vi "UHR-Fleezers Control (host) -Leonardo 04-2018 V2.vi"(0 "Tab Control":T5(tab)=enum."Trap Control (RF)") -> ()   [LabVIEW 2013] (continued)
                      n1370 = Not(x="Limits Enable") -> (.not. x?=w2097:bool)
                      n1371 = Or(x=w2098, y=w2097) -> (x .or. y?=w2099:bool)
                      n1372 = case shown="True" w2099 {
                        tunnel: w2106 -> [_ w2139]
                        tunnel: w2105 -> [_ w2130]
                        tunnel: w2095 -> [_ w2137]
                        tunnel: w2104 -> [_ w2136]
                        tunnel: w2093 -> [_ w2135]
                        tunnel: w2103 -> [_ w2134]
                        tunnel: w2088 -> [_ w2132]
                        tunnel: w2087 -> [_ w2131]
                        frame False {
                        }
                        frame True {
                          n1373 = local read "BD 1 Frequency 3 (MHz)"() -> (w2138:dbl)
                          n1374 = local read "BD 2 Frequency 3 (MHz)"() -> (w2133:dbl)
                          n1375 = local write "Trap Delta (MHz)"(w2130) -> ()
                          n1376 = property on="Initial delta (MHz)" class="DigNum (strict)"("Val(Sgnl)"=w2130) -> ()  [unwired: 2 in, 2 out]
                          n1377 = call "set RF board frequency - interlace.vi"("Board 2 Frequency Limits"=w2131, "Board 1 Frequency Limits"=w2132, "FPGA VI Reference In"=w2139, "Board 2 Frequency 3 (MHz)"=w2133, "Board 1 Frequency 3 (MHz)"=w2138, "Board 2 Frequency 2 (MHz)"=w2134, "Board 2 Frequency 1 (MHz)"=w2135, "Board 1 Frequency 2 (MHz)"=w2136, "Board 1 Frequency 1  (MHz)"=w2137) -> ()  [unwired: 1 in, 2 out]
                          n1378 = local write "BD 2 Frequency 1 (MHz)"(w2135) -> ()
                          n1379 = local write "BD 1 Frequency 1 (MHz)"(w2137) -> ()
                        }
                      }
                    }
                    frame True {
                    }
                  }
                }
                event Mouse Up {
                  n1380 = event-data() -> ("Button"=w2140:u16)  [unwired: 8 out]
                  n1381 = case shown="3" w2140 {
                    tunnel: [FALSE TRUE] -> w2141
                    frame 0, Default {
                    }
                    frame 3 {
                      n1382 = local write "Manipulating Trap"(FALSE ("Manipulating Trap")) -> ()
                    }
                  }
                }
              }
            }
          }
        }
      }
      event Mouse Move {
        n1383 = event-data() -> ()  [unwired: 6 out]
      }
    }
    n1384 = local read "Stop All"() -> (w1962:bool)
    n1385 = node-c288() -> ()  [unwired: 2 out]
  }
  n1386 = node-c288(w47) -> ()  [unwired: 1 out]
  n1387 = node-c288(w96) -> ()  [unwired: 1 out]
  n1388 = node-c288(w103) -> ()  [unwired: 1 out]
  n1389 = node-c288(i64 1 ("Period"), 1 ("Processor")) -> (w188:T25)  [unwired: 2 out]
  n1390 = timed-loop "Acquire Data" {
    tunnel: w55 -> [w2450]
    tunnel: w70 -> [w2449]
    tunnel: [w2480] -> w63
    tunnel: [w2474] -> w62
    timing: w188 -> [_]
    timing-out: [_] -> w187
    tunnel: w89 -> [w2296]
    stop <- "Stop All" stop-if-true
    (unwired) u32 0 ("Number of Elements")
    w2283 = "NI_ChannelName" ("name")
    n1391 = node-c288() -> ()  [unwired: 2 out]
    n1392 = First Call?() -> (First Call?: T/F=w2249:bool)
    n1393 = Or(x="Reset", y=w2249) -> (x .or. y?=w2250:bool)
    n1394 = local read "MCL Tracking"() -> (w2187:bool)
    n1395 = case "Reset data stream" shown="True" w2250 {
      tunnel: w2450 -> [w2600 w2608]
      tunnel: w2449 -> [w2599 w2607]
      tunnel: [w2600 w2602] -> w2185
      tunnel: [w2599 w2601] -> w2445
      frame False {
      }
      frame True {
        w2605 = TRUE ("AI to FIFO")
        n1396 = local write "Overflow (data lost)"(FALSE ("Overflow (data lost)")) -> ()
        n1397 = call "reset FPGA DMA.vi"("error in"=w2607, "FPGA VI Reference In"=w2608) -> ("error out"=w2603:errorcluster, "FPGA VI Reference Out"=w2604:T20)
        n1398 = xnode "Read/Write Control"("FPGA VI Reference In"=w2604, "error in"=w2603, "AI to FIFO"=w2605, "APD to FIFO"=w2605) -> ("FPGA VI Reference Out"=w2602:T20, "error out"=w2601:errorcluster)
      }
    }
    n1399 = Or(x="Start AOD Scan", y="Trap Raster Scan") -> (x .or. y?=w2403:bool)
    n1400 = case "Start AOM raster scan" shown="True" w2403 {
      tunnel: w2185 -> [w3341 w3352]
      tunnel: w2445 -> [w3340 w3351]
      tunnel: [w3341 w3345] -> w2184
      tunnel: [w3340 w3344] -> w2444
      frame False {
      }
      frame True {
        n1401 = case shown="True" "Restart DMA? (AOD)" {
          tunnel: [w3392 w3394] -> w3346
          tunnel: [w3391 w3393] -> w3347
          tunnel: w3352 -> [w3392 w3396]
          tunnel: w3351 -> [w3391 w3395]
          frame False {
          }
          frame True {
            n1402 = local write "Overflow (data lost)"(FALSE ("Overflow (data lost)")) -> ()
            n1403 = call "reset FPGA DMA.vi"("error in"=w3395, "FPGA VI Reference In"=w3396) -> ("error out"=w3393:errorcluster, "FPGA VI Reference Out"=w3394:T20)
          }
        }
        n1404 = local write "Trap Raster Scan"(FALSE ("Trap Raster Scan")) -> ()
        n1405 = case shown="False" "Move MCL Also?" {
          tunnel: w3347 -> [w3356 w3386]
          tunnel: w3346 -> [w3357 w3387]
          tunnel: [w3355 w3390] -> w3345
          tunnel: [w3354 w3389] -> w3344
          tunnel: "Raster to target force?" -> [w3353 w3359]
          frame False {
            w3358 = TRUE ("AI to FIFO")
            n1406 = xnode "Read/Write Control"("FPGA VI Reference In"=w3357, "error in"=w3356, "AI to FIFO"=w3358, "APD to FIFO"=w3358, "Start scan"=w3358, "Raster to target force"=w3353) -> ("FPGA VI Reference Out"=w3355:T20, "error out"=w3354:errorcluster)
          }
          frame True {
            w3383 = FALSE ("1D or 2D Scan?")
            w3388 = TRUE ("AI to FIFO")
            # "Count for MCL loop"
            # "N total cycles"
            # "N steps"
            # "V_int"
            n1407 = local read "Scan Range (nm)"() -> (w3365:dbl)
            n1408 = local read "Number of F/B Scans (AOD)"() -> (w3382:u16)
            n1409 = Sign(1:w3365) -> (0:w3364:dbl)
            n1410 = Compound Arithmetic op=MULTIPLY(w3365, "MCL Step Position Ratio", "MCL/AOM Scale Tweak") -> (w3369:dbl)
            n1411 = Negate(x=w3364) -> (-x=w3361:dbl)
            n1412 = Multiply(x=w3361, y="MCL Step Increment (V_int)") -> (x*y=w3363:dbl)
            n1413 = Divide(x=w3369, y="MCL X Cal (nm/V)") -> (x/y=w3375:dbl)
            n1414 = Multiply(x=32767.0 ("y"), y=w3375) -> (x*y=w3381:dbl)
            n1415 = local read "Total Counts (ticks)"() -> (w3366:u32)
            n1416 = local read "Cycles/step (AOD)"() -> (w3377:u64)
            n1417 = local read "Scan steps (AOD)"() -> (w3378:u64)
            n1418 = Divide(x=w3381, y=10.0) -> (x/y=w3374:dbl)
            n1419 = Divide(x=w3374, y="MCL Step Increment (V_int)") -> (x/y=w3372:dbl)
            n1420 = Absolute Value(x=w3372) -> (abs(x)=w3360:dbl)
            n1421 = Compound Arithmetic op=MULTIPLY(w3378, w3377, w3366) -> (w3373:u64)
            n1422 = local write "wait to reset values"(w3388) -> ()
            n1423 = local write "MCL Scanning"(w3388) -> ()
            n1424 = Divide(x=w3373, y=w3360) -> (x/y=w3370:dbl)
            "MCL Count" <- w3370
            n1425 = xnode "Read/Write Control"("FPGA VI Reference In"=w3387, "error in"=w3386, "Scan steps (MCL)"=w3360, "Number of scans (MCL)"=w3382, "Cycles per step (MCL)"=u64 1, "Scan freq.  increment (MCL)"=w3363, "1D or 2D Scan?"=w3383, "MCL Scan Axis"=w3383, "Cont. Scan (MCL)"=w3383, "MCL count"=w3370) -> ("FPGA VI Reference Out"=w3385:T20, "error out"=w3384:errorcluster)
            n1426 = xnode "Read/Write Control"("FPGA VI Reference In"=w3385, "error in"=w3384, "AI to FIFO"=w3388, "APD to FIFO"=w3388, "Start scan"=w3388, "Start scan (MCL)"=w3388, "Raster to target force"=w3359) -> ("FPGA VI Reference Out"=w3390:T20, "error out"=w3389:errorcluster)
          }
        }
        "Raster Scanning..." <- TRUE ("Scanning...")
      }
    }
    n1427 = And(x="Save scans", y=w2403) -> (x .and. y?=w2443:bool)
    n1428 = Compound Arithmetic op=OR("Start MCL Scan", "Confocal Image", "Confocal Linescan") -> (w2401:bool)
    n1429 = And(x="Save Data (MCL)", y=w2401) -> (x .and. y?=w2442:bool)
    n1430 = case "Start MCL raster scan" shown="True" w2401 {
      tunnel: w2184 -> [w2893 w2908]
      tunnel: w2444 -> [w2892 w2907]
      tunnel: [w2893 w2903] -> w2219
      tunnel: [w2892 w2902] -> w2218
      tunnel: [FALSE w2901] -> w2428
      tunnel: "Start MCL Scan" -> [_ w2896]
      tunnel: "Confocal Image" -> [_ w2895]
      tunnel: "Confocal Linescan" -> [_ _]
      frame False {
      }
      frame True {
        w2901 = TRUE
        n1431 = case shown="True" "Restart DMA? (MCL)" {
          tunnel: [w2953 w2955] -> w2906
          tunnel: [w2952 w2954] -> w2905
          tunnel: w2908 -> [w2953 w2958]
          tunnel: w2907 -> [w2952 w2957]
          frame False {
          }
          frame True {
            n1432 = call "reset FPGA DMA.vi"("error in"=w2957, "FPGA VI Reference In"=w2958) -> ("error out"=w2954:errorcluster, "FPGA VI Reference Out"=w2955:T20)
            n1433 = local write "Overflow (data lost)"(FALSE ("Overflow (data lost)")) -> ()
          }
        }
        n1434 = case shown="False" w2896 {
          selector: w2896 -> [_ w2912]
          tunnel: w2895 -> [w2911 _]
          tunnel: [w2911 w2912] -> w2894
          frame False {
            n1435 = property on="2D or 1D Scan" class="Bool (strict)"("Val(Sgnl)"=w2911) -> ()  [unwired: 2 in, 2 out]
            n1436 = property on="Confocal Image" class="Bool (strict)"("Value"=FALSE ("Start Confocal Map")) -> ()  [unwired: 2 in, 2 out]
          }
          frame True {
          }
        }
        n1437 = local write "MCL Scanning"(w2901) -> ()
        n1438 = local read "AO1"() -> (w2898:dbl)
        n1439 = local read "AO2"() -> (w2897:dbl)
        n1440 = case shown="True" "Center Scan" {
          tunnel: w2906 -> [w2919 w2951]
          tunnel: w2905 -> [w2918 w2950]
          tunnel: [w2917 w2949] -> w2903
          tunnel: [w2916 w2948] -> w2902
          tunnel: [w2914 w2935] -> w2900
          tunnel: [w2913 w2934] -> w2899
          tunnel: w2898 -> [w2914 w2940]
          tunnel: w2897 -> [w2913 w2943]
          tunnel: w2894 -> [_ _]
          frame False {
            w2915 = TRUE ("AI to FIFO")
            n1441 = xnode "Read/Write Control"("FPGA VI Reference In"=w2919, "error in"=w2918, "AI to FIFO"=w2915, "APD to FIFO"=w2915, "Start scan (MCL)"=w2915) -> ("FPGA VI Reference Out"=w2917:T20, "error out"=w2916:errorcluster)
          }
          frame True {
            w2947 = TRUE ("AI to FIFO")
            n1442 = local read "Scan steps (MCL)"() -> (w2926:u64)
            n1443 = local read "Scan lines (y)"() -> (w2922:u64)
            n1444 = local read "Fast Scan Dir"() -> (w2933:bool)
            n1445 = local read "Actual MCL Inc (V)"() -> (w2923:dbl)
            n1446 = Decrement(x=w2922) -> (x-1=w2921:u64)
            n1447 = Decrement(x=w2926) -> (x-1=w2925:u64)
            n1448 = Multiply(x=w2923, y=w2921) -> (x*y=w2920:dbl)
            n1449 = Divide(x=w2920, y=2.0) -> (x/y=w2930:dbl)
            n1450 = Multiply(x=w2923, y=w2925) -> (x*y=w2924:dbl)
            n1451 = Divide(x=w2924, y=2.0) -> (x/y=w2929:dbl)
            n1452 = Select(t=w2929, s=w2933, f=w2930) -> (s? t:f=w2928:dbl)
            n1453 = Select(t=w2930, s=w2933, f=w2929) -> (s? t:f=w2932:dbl)
            n1454 = Subtract(x=w2940, y=w2932) -> (x-y=w2931:dbl)
            n1455 = Subtract(x=w2943, y=w2928) -> (x-y=w2927:dbl)
            n1456 = local read "2D or 1D Scan"() -> (w2945:bool)
            n1457 = Not(x=w2933) -> (.not. x?=w2939:bool)
            n1458 = Not(x=w2945) -> (.not. x?=w2941:bool)
            n1459 = And(x=w2933, y=w2941) -> (x .and. y?=w2942:bool)
            n1460 = And(x=w2941, y=w2939) -> (x .and. y?=w2944:bool)
            n1461 = Select(t=w2943, s=w2944, f=w2927) -> (s? t:f=w2934:dbl)
            n1462 = Select(t=w2940, s=w2942, f=w2931) -> (s? t:f=w2935:dbl)
            n1463 = call "Volt to I16.vi"("Voltage In"=w2935) -> ("I16 Voltage Out"=w2938:i16)
            n1464 = call "Volt to I16.vi"("Voltage In"=w2934) -> ("I16 Voltage Out"=w2937:i16)
            n1465 = xnode "Read/Write Control"("FPGA VI Reference In"=w2951, "error in"=w2950, "AI to FIFO"=w2947, "APD to FIFO"=w2947, "Start scan (MCL)"=w2947, "AO1 (Y)"=w2938, "AO2 (X)"=w2937) -> ("FPGA VI Reference Out"=w2949:T20, "error out"=w2948:errorcluster)
          }
        }
        "Initial Y" <- w2900
        "Initial X" <- w2899
        "wait to reset values" <- w2901
      }
    }
    n1466 = local read "Trap Pos Elements/DMA read"() -> (w2292:u32)
    n1467 = local read "Trap AI Elements/DMA read"() -> (w2217:u32)
    n1468 = local read "APD Elements/DMA read"() -> (w2331:u32)
    n1469 = local read "Trap AI FIFO Depth"() -> (w2490:u32)
    n1470 = xnode "Invoke Method"("FPGA VI Reference In"=w2219, "error in"=w2218, "Number of Elements"=w2292, "Timeout (ms)"=-1) -> ("Data"=w2256:u16[], "Elements Remaining"=→"Trap Pos FIFO El Remaining":u32)  [unwired: 2 out]
    n1471 = xnode "Invoke Method"("FPGA VI Reference In"=w2219, "error in"=w2218, "Number of Elements"=w2217, "Timeout (ms)"=-1 ("Timeout")) -> ("FPGA VI Reference Out"=w2188:T20, "error out"=w2220:errorcluster, "Data"=w2216:i16[], "Elements Remaining"=w2221:u32)
    "Trap AI FIFO El. Rem." <- w2221
    n1472 = xnode "Get APD Data"("FPGA VI Reference In"=w2219, "error in"=w2218, "Number of Elements"=w2331, "Timeout (ms)"=-1) -> ("Data"=w2330:u32[], "Elements Remaining"=→"APD FIFO Elements Remaining":u32)  [unwired: 2 out]
    n1473 = Subtract(x=w2490, y=w2217) -> (x-y=w2489:u32)
    n1474 = Decimate 1D Array(w2256) -> (w2253:u16[], w2255:u16[], w2254:u16[])
    n1475 = Divide(x=w2221, y=w2489) -> (x/y=w2488:dbl)
    "Buffer Status" <- w2488
    n1476 = To Unsigned Long Integer(number=w2253) -> (unsigned 32bit integer=w2252:u32[])
    n1477 = Join Numbers(hi=w2255, lo=w2254) -> ((hi.lo)=w2251:u32[])
    n1478 = Equal?(x=w2488, y=1.0) -> (x = y?=w2486:bool)
    n1479 = Join Numbers(hi=w2252, lo=w2251) -> ((hi.lo)=w2245:u64[])
    n1480 = call "IR AOM word to freq - vec.vi"("Frequency Word In (double vec)"=w2245) -> ("Frequency Out"=w2291:dbl[])
    n1481 = case "Alert buffer overflow" shown="True" w2486 {
      frame False {
      }
      frame True {
        n1482 = call <vilib>:"Beep.vi"() -> ()  [unwired: 3 in, 9 out]
        "Overflow (data lost)" <- TRUE ("Overflow (data lost)")
      }
    }
    n1483 = Decimate 1D Array(w2291) -> (w2290:dbl[], w2289:dbl[])
    n1484 = Array Size(array=w2216) -> (size(s)=→"Waveform Chart":i32)
    n1485 = Build Array(w2290, w2289) -> (w2288:dbl[][])
    n1486 = local read "Trap Sets"() -> (w2363:u32)
    n1487 = case "Deinterlace trap data, average down PSD" shown="2" w2363 {
      tunnel: w2216 -> [w2988 w3053]
      tunnel: [w2985 w3050] -> w2356
      tunnel: [w2988 w3052] -> w2248
      tunnel: "Detector Type" -> [w2987 w3048]
      tunnel: [w2986 w3051] -> w2355
      tunnel: [w2984 w3049] -> w2461
      frame 1, Default {
        n1488 = Divide(x=w2988, y=3276.7) -> (x/y=w2989:dbl[])
        n1489 = Decimate 1D Array(w2989) -> (w2998:dbl[], w2997:dbl[], w2996:dbl[], w2995:dbl[], w2994:dbl[], w2993:dbl[], w2992:dbl[], w2991:dbl[])
        n1490 = case shown="\"IR-QPD + PSD + FB-QPD position\"" w2987 {
          tunnel: w2998 -> [w3022 w3047]
          tunnel: w2997 -> [w3021 w3046]
          tunnel: w2996 -> [w3006 w3024]
          tunnel: w2995 -> [w3007 w3034]
          tunnel: w2994 -> [w3020 w3045]
          tunnel: w2993 -> [w3019 w3044]
          tunnel: w2992 -> [w3003 w3025]
          tunnel: w2991 -> [w3002 w3023]
          tunnel: [w3001 w3031] -> w2986
          tunnel: [w3000 w3030] -> w2985
          tunnel: [w2999 w3029] -> w2984
          frame "IR-QPD + PSD + FB-QPD", Default {
            w2999 = 0  # Channel pattern
            n1491 = Divide(x=w3022, y=w3007) -> (x/y=w3009:dbl[])
            n1492 = Divide(x=w3021, y=w3007) -> (x/y=w3008:dbl[])
            n1493 = Divide(x=w3020, y=w3003) -> (x/y=w3005:dbl[])
            n1494 = Divide(x=w3019, y=w3002) -> (x/y=w3004:dbl[])
            n1495 = Build Array(w3009, w3008, w3007, w3006, w3005, w3004, w3003, w3002) -> (w3000:dbl[][])
            n1496 = Bundle("T1 Y", "T1 X", "T1 Sum", "FB Sum", "PSD Y", "PSD X", "PSD Y Sum", "PSD X Sum") -> (w3018:T42)  [unwired: 1 out]
            n1497 = Cluster To Array(cluster=w3018) -> (array=w3001:string[])
          }
          frame "IR-QPD + PSD + FB-QPD position" {
            w3029 = 3  # Channel pattern
            n1498 = Negate(x=w3025) -> (-x=w3026:dbl[])
            n1499 = Divide(x=w3047, y=w3034) -> (x/y=w3036:dbl[])
            n1500 = Divide(x=w3046, y=w3034) -> (x/y=w3035:dbl[])
            n1501 = Divide(x=w3045, y=w3025) -> (x/y=w3033:dbl[])
            n1502 = Divide(x=w3044, y=w3026) -> (x/y=w3032:dbl[])
            n1503 = Build Array(w3036, w3035, w3034, w3023, w3024, w3033, w3032, w3025) -> (w3030:dbl[][])
            n1504 = Bundle("T1 Y", "T1 X", "T1 Sum", "FB X", "FB Sum", "PSD Y", "PSD X", "PSD Y Sum") -> (w3043:T42)  [unwired: 1 out]
            n1505 = Cluster To Array(cluster=w3043) -> (array=w3031:string[])
          }
        }
      }
      frame 2 {
        n1506 = case shown="\"UCB Fleezers 052511\"" w3048 {
          tunnel: w3053 -> [w3115 w3182 w3214 w3319]
          tunnel: [w3054 w3174 w3210 w3250] -> w3052
          tunnel: [w3081 w3165 w3212 w3297] -> w3051
          tunnel: [w3080 w3129 w3201 w3264] -> w3050
          tunnel: [w3074 w3164 w3249 w3295] -> w3049
          frame "IR-QPD + PSD + FB-QPD", Default {
            w3074 = 1  # Channel pattern
            # "time average x2 the 4th signal and the 4 psd signals (detection laser)"
            # "deinterlace 3 signals from qpd"
            n1507 = Decimate 1D Array(w3115) -> (w3114:i16[], w3113:i16[], w3079:i16[], w3112:i16[], w3102:i16[], w3100:i16[], w3099:i16[], w3097:i16[])
            n1508 = call "downsample 1D array - double.vi"("Ave N"=2.0, "Array In"=w3102) -> ("Array Out"=w3101:dbl[])  [unwired: 1 out]
            n1509 = call "downsample 1D array - double.vi"("Ave N"=2.0, "Array In"=w3097) -> ("Array Out"=w3096:dbl[])  [unwired: 1 out]
            n1510 = call "downsample 1D array - double.vi"("Ave N"=2.0, "Array In"=w3099) -> ("Array Out"=w3098:dbl[])  [unwired: 1 out]
            n1511 = call "downsample 1D array - double.vi"("Ave N"=2.0, "Array In"=w3100) -> ("Array Out"=w3082:dbl[])  [unwired: 1 out]
            n1512 = Decimate 1D Array(w3114) -> (w3111:i16[], w3083:i16[])
            n1513 = Decimate 1D Array(w3113) -> (w3110:i16[], w3108:i16[])
            n1514 = Decimate 1D Array(w3112) -> (w3109:i16[], w3107:i16[])
            n1515 = Decimate 1D Array(w3079) -> (w3078:i16[], w3077:i16[])
            n1516 = Interleave 1D Arrays(w3111, w3110, w3109, w3083, w3108, w3107, w3078, w3077, w3101, w3082, w3098, w3096) -> (w3095:dbl[])
            n1517 = To Word Integer(number=w3095) -> (16bit integer=w3054:i16[])
            n1518 = Divide(x=w3095, y=3276.7) -> (x/y=w3094:dbl[])
            n1519 = Decimate 1D Array(w3094) -> (w3093:dbl[], w3092:dbl[], w3091:dbl[], w3090:dbl[], w3089:dbl[], w3088:dbl[], w3076:dbl[], w3075:dbl[], w3087:dbl[], w3086:dbl[], w3085:dbl[], w3084:dbl[])
            n1520 = Divide(x=w3093, y=w3091) -> (x/y=w3061:dbl[])
            n1521 = Divide(x=w3092, y=w3091) -> (x/y=w3060:dbl[])
            n1522 = Divide(x=w3090, y=w3088) -> (x/y=w3059:dbl[])
            n1523 = Divide(x=w3089, y=w3088) -> (x/y=w3058:dbl[])
            n1524 = Divide(x=w3087, y=w3085) -> (x/y=w3057:dbl[])
            n1525 = Divide(x=w3086, y=w3084) -> (x/y=w3056:dbl[])
            n1526 = Bundle("T1 Y", "T1 X", "T1 Sum", "T2 Y", "T2 X", "T2 Sum", "T1 FB Sum", "T2 FB Sum", "PSD Y", "PSD X", "PSD Y Sum", "PSD X Sum") -> (w3062:T43)  [unwired: 1 out]
            n1527 = Build Array(w3061, w3060, w3091, w3059, w3058, w3088, w3076, w3075, w3057, w3056, w3085, w3084) -> (w3080:dbl[][])
            n1528 = Cluster To Array(cluster=w3062) -> (array=w3081:string[])
          }
          frame "IR-QPD + PSD + FB-QPD X position" {
            w3164 = 2  # Channel pattern
            # "convert\nADC numbers\nto volts"
            # "time average x2 the 3 psd signals (detection laser)"
            # "deinterlace 3 signals from qpds"
            n1529 = Decimate 1D Array(w3182) -> (w3181:i16[], w3180:i16[], w3117:i16[], w3118:i16[], w3127:i16[], w3124:i16[], w3121:i16[], w3152:i16[])
            n1530 = Decimate 1D Array(w3181) -> (w3179:i16[], w3166:i16[])
            n1531 = call "downsample 1D array - I16.vi"("Ave N"=2.0, "Array In"=w3127) -> ("Array Out"=w3125:i16[])  [unwired: 1 in]
            n1532 = call "downsample 1D array - I16.vi"("Ave N"=2.0, "Array In"=w3124) -> ("Array Out"=w3122:i16[])  [unwired: 1 in]
            n1533 = Decimate 1D Array(w3180) -> (w3178:i16[], w3176:i16[])
            n1534 = Decimate 1D Array(w3118) -> (w3177:i16[], w3175:i16[])
            n1535 = Decimate 1D Array(w3152) -> (w3151:i16[], w3149:i16[])
            n1536 = Decimate 1D Array(w3117) -> (w3150:i16[], w3148:i16[])
            n1537 = call "downsample 1D array - I16.vi"("Ave N"=2.0, "Array In"=w3121) -> ("Array Out"=w3119:i16[])  [unwired: 1 in]
            n1538 = Interleave 1D Arrays(w3179, w3178, w3177, w3166, w3176, w3175, w3151, w3150, w3149, w3148, w3125, w3122, w3119) -> (w3174:i16[])
            n1539 = Divide(x=w3174, y=3276.7) -> (x/y=w3173:dbl[])
            n1540 = Decimate 1D Array(w3173) -> (w3172:dbl[], w3171:dbl[], w3170:dbl[], w3169:dbl[], w3168:dbl[], w3167:dbl[], w3140:dbl[], w3138:dbl[], w3137:dbl[], w3135:dbl[], w3134:dbl[], w3133:dbl[], w3130:dbl[])
            n1541 = Divide(x=w3172, y=w3170) -> (x/y=w3156:dbl[])
            n1542 = Divide(x=w3171, y=w3170) -> (x/y=w3155:dbl[])
            n1543 = Divide(x=w3169, y=w3167) -> (x/y=w3154:dbl[])
            n1544 = Divide(x=w3168, y=w3167) -> (x/y=w3153:dbl[])
            n1545 = Divide(x=w3140, y=w3138) -> (x/y=w3139:dbl[])
            n1546 = Divide(x=w3137, y=w3135) -> (x/y=w3136:dbl[])
            n1547 = Divide(x=w3134, y=w3130) -> (x/y=w3132:dbl[])
            n1548 = Negate(x=w3130) -> (-x=w3128:dbl[])
            n1549 = Divide(x=w3133, y=w3128) -> (x/y=w3131:dbl[])
            n1550 = Bundle("T1 Y", "T1 X", "T1 Sum", "T2 Y", "T2 X", "T2 Sum", "T1 FB X", "T1 FB Sum", "T2 FB X", "T2 FB Sum", "PSD Y", "PSD X", "PSD Y Sum") -> (w3157:T44)  [unwired: 1 out]
            n1551 = Build Array(w3156, w3155, w3170, w3154, w3153, w3167, w3139, w3138, w3136, w3135, w3132, w3131, w3130) -> (w3129:dbl[][])
            n1552 = Cluster To Array(cluster=w3157) -> (array=w3165:string[])
          }
          frame "UCB Fleezers 052511" {
            w3249 = 2  # Channel pattern
            n1553 = Decimate 1D Array(w3214) -> (w3247:i16[], w3246:i16[], w3195:i16[], w3213:i16[], w3187:i16[], w3209:i16[], w3208:i16[], w3192:i16[])
            n1554 = Decimate 1D Array(w3247) -> (w3245:i16[], w3232:i16[])
            n1555 = Decimate 1D Array(w3246) -> (w3244:i16[], w3243:i16[])
            n1556 = Decimate 1D Array(w3195) -> (w3189:i16[], w3188:i16[])
            n1557 = Decimate 1D Array(w3213) -> (w3194:i16[], w3193:i16[])
            n1558 = call "downsample 1D array - I16.vi"("Ave N"=2.0, "Array In"=w3187) -> ("Array Out"=w3186:i16[])  [unwired: 1 in]
            n1559 = Decimate 1D Array(w3192) -> (w3191:i16[], w3190:i16[])
            n1560 = call "downsample 1D array - I16.vi"("Ave N"=2.0, "Array In"=w3208) -> ("Array Out"=w3184:i16[])  [unwired: 1 in]
            n1561 = call "downsample 1D array - I16.vi"("Ave N"=2.0, "Array In"=w3209) -> ("Array Out"=w3185:i16[])  [unwired: 1 in]
            n1562 = Interleave 1D Arrays(w3245, w3244, w3194, w3232, w3243, w3193, w3191, w3189, w3190, w3188, w3186, w3185, w3184) -> (w3210:i16[])
            n1563 = Divide(x=w3210, y=3276.7) -> (x/y=w3239:dbl[])
            n1564 = Decimate 1D Array(w3239) -> (w3238:dbl[], w3237:dbl[], w3236:dbl[], w3235:dbl[], w3234:dbl[], w3233:dbl[], w3207:dbl[], w3205:dbl[], w3204:dbl[], w3202:dbl[], w3200:dbl[], w3197:dbl[], w3198:dbl[])
            n1565 = Divide(x=w3238, y=w3236) -> (x/y=w3219:dbl[])
            n1566 = Divide(x=w3237, y=w3236) -> (x/y=w3218:dbl[])
            n1567 = Divide(x=w3235, y=w3233) -> (x/y=w3217:dbl[])
            n1568 = Divide(x=w3234, y=w3233) -> (x/y=w3216:dbl[])
            n1569 = Divide(x=w3207, y=w3205) -> (x/y=w3206:dbl[])
            n1570 = Divide(x=w3204, y=w3202) -> (x/y=w3203:dbl[])
            n1571 = Divide(x=w3200, y=w3198) -> (x/y=w3199:dbl[])
            n1572 = Divide(x=w3197, y=w3198) -> (x/y=w3196:dbl[])
            n1573 = Build Array(w3219, w3218, w3236, w3217, w3216, w3233, w3206, w3205, w3203, w3202, w3199, w3196, w3198) -> (w3201:dbl[][])
            n1574 = Bundle("T1 Y", "T1 X", "T1 Sum", "T2 Y", "T2 X", "T2 Sum", "T1 FB X", "T2 FB Sum", "T2 FB X", "T2 FB Sum", "PSD Y", "PSD X", "PSD Sum") -> (w3220:T44)  [unwired: 1 out]
            n1575 = Cluster To Array(cluster=w3220) -> (array=w3212:string[])
          }
          frame "IR-QPD + PSD + FB-QPD XY positions" {
            w3295 = 4  # Channel pattern
            # "time average x2 the 3 psd signals (detection laser)"
            # "deinterlace 3 signals from qpds"
            n1576 = Decimate 1D Array(w3319) -> (w3318:i16[], w3317:i16[], w3296:i16[], w3316:i16[], w3262:i16[], w3308:i16[], w3307:i16[], w3284:i16[])
            n1577 = Decimate 1D Array "QPD Y"(w3318) -> (w3315:i16[], w3298:i16[])
            n1578 = call "downsample 1D array - double.vi"("Ave N"=2.0, "Array In"=w3308) -> ("Array Out"=w3283:dbl[])  [unwired: 1 out]
            n1579 = call "downsample 1D array - double.vi"("Ave N"=2.0, "Array In"=w3307) -> ("Array Out"=w3282:dbl[])  [unwired: 1 out]
            n1580 = Decimate 1D Array "Feedback Sum"(w3296) -> (w3280:i16[], w3278:i16[])
            n1581 = Decimate 1D Array "Feedback Y"(w3262) -> (w3261:i16[], w3260:i16[])
            n1582 = Decimate 1D Array "Feedback X"(w3284) -> (w3281:i16[], w3279:i16[])
            n1583 = Decimate 1D Array "QPD Sum"(w3316) -> (w3313:i16[], w3311:i16[])
            n1584 = Decimate 1D Array "QPD X"(w3317) -> (w3314:i16[], w3312:i16[])
            n1585 = Interleave 1D Arrays(w3315, w3314, w3313, w3298, w3312, w3311, w3261, w3281, w3280, w3260, w3279, w3278, w3283, w3282) -> (w3306:dbl[])
            n1586 = To Word Integer(number=w3306) -> (16bit integer=w3250:i16[])
            n1587 = Divide(x=w3306, y=3276.7) -> (x/y=w3305:dbl[])
            n1588 = Decimate 1D Array(w3305) -> (w3304:dbl[], w3303:dbl[], w3302:dbl[], w3301:dbl[], w3300:dbl[], w3299:dbl[], w3257:dbl[], w3271:dbl[], w3255:dbl[], w3256:dbl[], w3269:dbl[], w3253:dbl[], w3267:dbl[], w3265:dbl[])
            n1589 = Divide(x=w3304, y=w3302) -> (x/y=w3288:dbl[])
            n1590 = Divide(x=w3303, y=w3302) -> (x/y=w3287:dbl[])
            n1591 = Divide(x=w3301, y=w3299) -> (x/y=w3286:dbl[])
            n1592 = Divide(x=w3300, y=w3299) -> (x/y=w3285:dbl[])
            n1593 = Divide(x=w3257, y=w3255) -> (x/y=w3254:dbl[])
            n1594 = Divide(x=w3271, y=w3255) -> (x/y=w3270:dbl[])
            n1595 = Divide(x=w3256, y=w3253) -> (x/y=w3252:dbl[])
            n1596 = Divide(x=w3269, y=w3253) -> (x/y=w3268:dbl[])
            n1597 = Negate(x=w3265) -> (-x=w3263:dbl[])
            n1598 = Divide(x=w3267, y=w3263) -> (x/y=w3266:dbl[])
            n1599 = Bundle("T1 Y", "T1 X", "T1 Sum", "T2 Y", "T2 X", "T2 Sum", "T1 FB Y", "T1 FB X", "T1 FB Sum", "T2 FB Y", "T2 FB X", "T2 FB Sum", "PSD X", "PSD Y Sum") -> (w3251:T45)  [unwired: 1 out]
            n1600 = Build Array(w3288, w3287, w3302, w3286, w3285, w3299, w3254, w3270, w3255, w3252, w3268, w3253, w3266, w3265) -> (w3264:dbl[][])
            n1601 = Cluster To Array(cluster=w3251) -> (array=w3297:string[])
          }
        }
      }
    }
    "AI labels" <- w2355
    n1602 = xnode "Read/Write Control"("FPGA VI Reference In"=w2188) -> ("FPGA VI Reference Out"=w2181:T20, "BD1 Frequency Out 1"=w2202:u64)  [unwired: 1 in, 1 out]
    n1603 = local read "BD 1 Frequency 2 (MHz)"() -> (w2193:dbl)
    n1604 = To Double Precision Float(number=w2202) -> (double precision float=w2199:dbl)
    n1605 = Multiply(x=49125000.0, y=6.0) -> (x*y=w2198:dbl)
    n1606 = Multiply(x=w2199, y=w2198) -> (x*y=w2196:dbl)
    n1607 = Scale By Power Of 2(n=-48, x=w2196) -> (x*2^n=w2195:dbl)
    n1608 = local read "Dynamic Force FB"() -> (w2192:bool)
    n1609 = local read "Trap Pos. FB ON"() -> (w2191:bool)
    n1610 = Divide(x=w2195, y=1000000.0) -> (x/y=w2186:dbl)
    n1611 = case shown="True" w2187 {
      tunnel: w2186 -> [_ w2577]
      tunnel: w2184 -> [_ w2564]
      frame False {
      }
      frame True {
        n1612 = local read "AOM X Cal (nm/MHz)"() -> (w2574:dbl)
        n1613 = local read "Zero T1 position"() -> (w2576:dbl)
        n1614 = Subtract(x=w2577, y=w2576) -> (x-y=w2575:dbl)
        n1615 = Multiply(x=w2575, y=w2574) -> (x*y=w2573:dbl)
        n1616 = local read "MCL X Cal (nm/V)"() -> (w2570:dbl)
        n1617 = Multiply(x=w2573, y="Tracking factor") -> (x*y=w2571:dbl)
        n1618 = local read "Zero MCL x position"() -> (w2569:dbl)
        n1619 = Divide(x=w2571, y=w2570) -> (x/y=w2568:dbl)
        n1620 = Add(x=w2569, y=w2568) -> (x+y=w2561:dbl)
        "Current MCL (V)" <- w2561
        n1621 = Multiply(x=w2561, y=32767.0) -> (x*y=w2565:dbl)
        n1622 = Divide(x=w2565, y=10.0) -> (x/y=w2562:dbl)
        n1623 = To Word Integer(number=w2562) -> (16bit integer=w2563:i16)
        n1624 = xnode "Read/Write Control"("FPGA VI Reference In"=w2564, "AO2 (X)"=w2563) -> ()  [unwired: 1 in, 2 out]
      }
    }
    n1625 = Subtract(x=w2193, y=w2186) -> (x-y=w2182:dbl)
    "Current deltaFreq" <- w2182
    n1626 = Compound Arithmetic op=AND(w2192, w2191, "Real time offset \ncorrection for setpoint") -> (w2189:bool)
    n1627 = case shown="True" w2189 {
      tunnel: w2182 -> [_ w2580]
      tunnel: w2181 -> [_ w2579]
      frame False {
      }
      frame True {
        n1628 = local read "T1 kappa_x (pN/nm)"() -> (w2588:dbl)
        n1629 = local read "T1 alpha_x (nm/V)"() -> (w2589:dbl)
        n1630 = local read "Negate offset difference"() -> (w2590:bool)
        n1631 = local read "Offset file step size"() -> (w2598:dbl)
        n1632 = Multiply(x="Target Force (pN)", y=2.0) -> (x*y=w2586:dbl)
        n1633 = local read "Setpoint offset\nCorrection values"() -> (w2595:dbl[])
        n1634 = Divide(x=w2580, y=w2598) -> (x/y=w2597:dbl)
        n1635 = Select(t=-1, s=w2590, f=1) -> (s? t:f=w2591:i32)
        n1636 = To Long Integer(number=w2597) -> (32bit integer=w2596:i32)
        n1637 = Multiply(x=w2589, y=w2588) -> (x*y=w2585:dbl)
        n1638 = Divide(x=w2586, y=w2585) -> (x/y=w2584:dbl)
        n1639 = Index Array(array=w2595, index=w2596) -> (element=w2594:dbl)
        n1640 = Multiply(x=w2591, y=w2594) -> (x*y=w2583:dbl)
        n1641 = Add(x=w2584, y=w2583) -> (x+y=w2582:dbl)
        n1642 = To Fixed-Point(number=w2582) -> (fixed-point=w2578:fxp<+/-,16,1>)  [unwired: 1 in]
        "Actual setpoint" <- w2578
        n1643 = xnode "Read/Write Control"("FPGA VI Reference In"=w2579, "Trap Pos. FB SP"=w2578) -> ()  [unwired: 1 in, 2 out]
      }
    }
    n1644 = case shown="True" "Take full offset\n data for display" {
      tunnel: [w2547 w2553] -> w2380
      tunnel: [w2546 w2552] -> w2378
      tunnel: w2182 -> [_ w2559]
      frame False {
        n1645 = Divide(x="T2 offset_x (mV)", y=1000.0) -> (x/y=w2546:dbl)
        n1646 = Divide(x="T1 offset_x (mV)", y=1000.0) -> (x/y=w2547:dbl)
      }
      frame True {
        n1647 = local read "Offset Values"() -> (w2560:T14)
        n1648 = local read "Offset file step size"() -> (w2558:dbl)
        n1649 = Unbundle By Name(w2560) -> ("Trap 1X offset"=w2555:dbl[], "Trap 2X offset"=w2554:dbl[])
        n1650 = Divide(x=w2559, y=w2558) -> (x/y=w2557:dbl)
        n1651 = To Long Integer(number=w2557) -> (32bit integer=w2556:i32)
        n1652 = Index Array(array=w2555, index=w2556) -> (element=w2553:dbl)
        n1653 = Index Array(array=w2554, index=w2556) -> (element=w2552:dbl)
      }
    }
    n1654 = Decimate 1D Array(w2330) -> (w2353:u32[], w2298:u32[])
    n1655 = local read "DMA Update Period (s)"() -> (w2364:dbl)
    n1656 = local read "BD 1 Frequency 2 (MHz)"() -> (w2240:dbl)
    n1657 = local read "BD 1 Frequency 1 (MHz)"() -> (w2241:dbl)
    n1658 = Build Array(w2353, w2298) -> (w2425:u32[][])
    n1659 = local read "Data Period (s)"() -> (w2343:dbl)
    n1660 = Decimate 1D Array(w2248) -> (w2271:i16[], w2270:i16[], w2268:i16[], w2267:i16[])  [unwired: 9 out]
    n1661 = To Double Precision Float(number=w2425) -> (double precision float=w2426:dbl[][])
    n1662 = local read "APD Integration Time (s)"() -> (w2311:dbl)
    n1663 = Divide(x=w2271, y=w2270) -> (x/y=w2272:dbl[])
    n1664 = Divide(x=w2268, y=w2267) -> (x/y=w2269:dbl[])
    n1665 = feedback #1(0.0) -> (w2285:dbl)
    n1666 = Add(x=w2364, y=w2285) -> (x+y=w2463:dbl)
    n1667 = feedback-in #1(w2463) -> ()
    n1668 = local read "AOM X Cal (nm/MHz)"() -> (w2238:dbl)
    n1669 = To Time Stamp(1:w2285) -> (0:w2284:timestamp)
    n1670 = Split 1D Array(array=w2272, index="N El. to Ave.") -> (second subarray=w2275:dbl[])  [unwired: 1 out]
    n1671 = Split 1D Array(array=w2269, index="N El. to Ave.") -> (second subarray=w2274:dbl[])  [unwired: 1 out]
    n1672 = local read "Trap X AI1 (DMA)"() -> (w2273:T13)
    n1673 = Multiply(x=w2343, y="Trap Disp. Downsample") -> (x*y=w2286:dbl)
    "Display Period (s)" <- w2286
    n1674 = Bundle("BD 1 Frequency 1 (MHz)"=w2241, "BD 1 Frequency 2 (MHz)"=w2240) -> (w2242:T46)  [unwired: 1 out]
    n1675 = for "Trap AI" {
      tunnel: [w2983] -> w2457 mode=indexing
      tunnel: w2284 -> [w2973]
      tunnel: "Trap Disp. Downsample" -> [w2981]
      tunnel: w2356 -> [w2979] mode=indexing
      tunnel: w2343 -> [w2978]
      tunnel: w2355 -> [w2977] mode=indexing
      tunnel: w2283 -> [w2976]
      tunnel: [w2975] -> w2322 mode=indexing
      tunnel: w2286 -> [w2974]
      n1676 = Bundle By Name("Y"=w2979, "dt"=w2978) -> (w2980:waveform(dbl))  [unwired: 1 out]
      n1677 = Set Waveform Attribute(5:w2977, 6:w2976, 7:w2980) -> (3:w2975:waveform(dbl))  [unwired: 1 in, 2 out]
      n1678 = call "downsample 1D array - double.vi"("Ave N"=w2981, "Array In"=w2979) -> ("Array Out"=w2982:dbl[])  [unwired: 1 out]
      n1679 = Bundle By Name(cluster=w2975, "t0"=w2973, "Y"=w2982, "dt"=w2974) -> (w2983:waveform(dbl))
    }
    n1680 = call-poly <vilib>:"Mean.vi"("X"=w2274) -> ("mean"=w2262:dbl)  [unwired: 1 out]
    n1681 = call-poly <vilib>:"Mean.vi"("X"=w2275) -> ("mean"=w2263:dbl)  [unwired: 1 out]
    n1682 = Cluster To Array(cluster=w2242) -> (array=w2239:dbl[])
    n1683 = Reciprocal(x=w2286) -> (1/x=→"Trap Disp. Freq. (Hz)":dbl)
    n1684 = local read "Data points/scans (MCL)"() -> (w2437:dbl)
    n1685 = To Fixed-Point(number=w2262) -> (fixed-point=w2260:fxp<+/-,16,1>)  [unwired: 1 in]
    n1686 = To Fixed-Point(number=w2263) -> (fixed-point=w2261:fxp<+/-,16,1>)  [unwired: 1 in]
    n1687 = Bundle("Trap 1 Pos.", "Trap 2 Pos.") -> (w2282:cluster{string, string})  [unwired: 1 out]
    n1688 = Bundle By Name(cluster=w2273, "Set 1"=w2261, "Set 2"=w2260) -> (→"Trap X AI1 (DMA)":T13)
    n1689 = Cluster To Array(cluster=w2282) -> (array=w2279:string[])
    n1690 = for "Trap Position" {
      tunnel: w2288 -> [w2621] mode=indexing
      tunnel: "Trap Disp. Downsample" -> [w2620]
      tunnel: w2286 -> [w2618]
      tunnel: w2284 -> [w2617]
      tunnel: w2283 -> [w2615]
      tunnel: w2279 -> [w2614] mode=indexing
      tunnel: [w2613] -> w2237 mode=indexing
      tunnel: w2239 -> [w2611] mode=indexing
      tunnel: w2238 -> [w2609]
      n1691 = call "downsample 1D array - double.vi"("Ave N"=w2620, "Array In"=w2621) -> ("Array Out"=w2619:dbl[])  [unwired: 1 out]
      n1692 = Subtract(x=w2619, y=w2611) -> (x-y=w2612:dbl[])
      n1693 = Multiply(x=w2609, y=w2612) -> (x*y=w2610:dbl[])
      n1694 = Bundle By Name("Y"=w2610, "dt"=w2618, "t0"=w2617) -> (w2616:waveform(dbl))  [unwired: 1 out]
      n1695 = Set Waveform Attribute(5:w2614, 6:w2615, 7:w2616) -> (3:w2613:waveform(dbl))  [unwired: 1 in, 2 out]
    }
    "Trap Positions" <- w2237
    n1696 = Bundle("APD 1", "APD 2") -> (w2456:cluster{string, string})  [unwired: 1 out]
    n1697 = Cluster To Array(cluster=w2456) -> (array=w2453:string[])
    n1698 = for "APD" {
      tunnel: w2426 -> [w2962] mode=indexing
      tunnel: w2311 -> [w2970]
      tunnel: [w2966] -> w2318 mode=indexing
      tunnel: "APD Disp. Scale" -> [w2967]
      tunnel: w2283 -> [w2965]
      tunnel: w2453 -> [w2964] mode=indexing
      tunnel: "APD Disp. Downsample" -> [w2960]
      tunnel: [w2963] -> w2452
      tunnel: w2284 -> [w2959]
      n1699 = call "integrate 1D array interval - double.vi"("Ave N"=w2960, "Array In"=w2962) -> ("Array Out"=w2961:dbl[])  [unwired: 1 out]
      n1700 = Multiply(x=w2970, y=w2960) -> (x*y=w2963:dbl)
      n1701 = Divide(x=w2961, y=w2967) -> (x/y=w2968:dbl[])
      n1702 = Bundle By Name("t0"=w2959, "Y"=w2968, "dt"=w2963) -> (w2969:waveform(dbl))  [unwired: 1 out]
      n1703 = Set Waveform Attribute(5:w2964, 6:w2965, 7:w2969) -> (3:w2966:waveform(dbl))  [unwired: 1 in, 2 out]
    }
    "APD Display Period (s)" <- w2452
    n1704 = Reciprocal(x=w2452) -> (1/x=→"APD Display Freq. (Hz)":dbl)
    n1705 = local read "Display Period (s)"() -> (w2342:dbl)
    n1706 = Increment(x=w2437) -> (x+1=w2438:dbl)
    n1707 = Index Array(array=w2237, index=0) -> (element=w2235:waveform(dbl))
    n1708 = To Double Precision Float(number=w2353) -> (double precision float=w2352:dbl[])
    n1709 = feedback #2(w2438) -> (w2441:dbl)
    n1710 = Select(t=0, s=w2428, f=w2441) -> (s? t:f=w2434:dbl)
    n1711 = Array Size(array=w2352) -> (size(s)=w2440:i32)
    n1712 = Add(x=w2440, y=w2434) -> (x+y=w2435:dbl)
    n1713 = Unbundle By Name(w2235) -> ("Y"=w2233:dbl[])
    n1714 = feedback #3(w2353) -> (w2424:u32[])
    n1715 = Build Array (concatenate)(w2424, w2353) -> (w2421:u32[])
    n1716 = feedback #4(w2298) -> (w2317:u32[])
    n1717 = Divide(x="Bead Sep. Int. Time (s)", y=w2342) -> (x/y=w2231:dbl)
    n1718 = Build Array (concatenate)(w2317, w2298) -> (w2316:u32[])
    n1719 = Greater?(x=w2435, y=w2437) -> (0:w2436:bool)
    n1720 = feedback #5(w2233) -> (w2234:dbl[])
    n1721 = Build Array (concatenate)(w2233, w2234) -> (w2232:dbl[])
    n1722 = Select(t=w2434, s=w2436, f=w2435) -> (s? t:f=w2433:dbl)
    n1723 = feedback-in #2(w2433) -> ()
    n1724 = Array Size(array=w2421) -> (size(s)=w2418:i32)
    n1725 = Array Size(array=w2353) -> (size(s)=w2420:i32)
    n1726 = local read "MCL Scanning"() -> (w2431:bool)
    n1727 = local read "APD Integration Time (s)"() -> (w2325:dbl)
    n1728 = Build Array (concatenate)(w2318, w2457) -> (w2320:waveform(dbl)[])
    "All Signals" <- w2320
    n1729 = Split 1D Array(array=w2232, index=w2231) -> (first subarray=w2225:dbl[])  [unwired: 1 out]
    n1730 = feedback-in #5(w2225) -> ()
    n1731 = Multiply(x=w2420, y="APD Ave N") -> (x*y=w2419:dbl)
    n1732 = Greater?(x=w2418, y=w2419) -> (0:w2422:bool)
    n1733 = Not(x=w2436) -> (.not. x?=w2430:bool)
    n1734 = To Double Precision Float(number=w2298) -> (double precision float=w2297:dbl[])
    n1735 = call-poly <vilib>:"Mean.vi"("X"=w2225) -> ("mean"=w2224:dbl)  [unwired: 1 out]
    "Mean T1 Position (nm)" <- w2224
    n1736 = Subtract(x=w2225, y=w2224) -> (x-y=w2230:dbl[])
    n1737 = Square(x=w2230) -> (x^2=w2229:dbl[])
    n1738 = And(x=w2430, y=w2431) -> (x .and. y?=w2432:bool)
    n1739 = call-poly <vilib>:"Mean.vi"("X"=w2229) -> ("mean"=w2228:dbl)  [unwired: 1 out]
    n1740 = case shown="True" w2422 {
      tunnel: w2421 -> [w2743 w2750]
      tunnel: [w2743 w2748] -> w2369
      tunnel: w2419 -> [_ w2745]
      tunnel: w2418 -> [_ w2749]
      tunnel: w2316 -> [w2742 w2747]
      tunnel: [w2742 w2744] -> w2313
      frame False {
      }
      frame True {
        n1741 = Subtract(x=w2749, y=w2745) -> (x-y=w2746:dbl)
        n1742 = Array Subset(array=w2750, index=w2746, length=w2745) -> (w2748:u32[])
        n1743 = Array Subset(array=w2747, index=w2746, length=w2745) -> (w2744:u32[])
      }
    }
    n1744 = feedback-in #3(w2369) -> ()
    n1745 = feedback-in #4(w2313) -> ()
    n1746 = Or(x=w2432, y=w2428) -> (x .or. y?=w2429:bool)
    n1747 = Square Root(x=w2228) -> (sqrt(x)=w2227:dbl)
    n1748 = Equal?(x="Tab Control 6", y=T36."High Res Display") -> (x = y?=w2359:bool)
    n1749 = Multiply(x="APD Disp. Scale", y=w2318) -> (x*y=w2327:waveform(dbl)[])
    n1750 = Multiply(x="APD Disp. Downsample", y=w2325) -> (x*y=w2323:dbl)
    n1751 = Multiply(x=10.0, y=w2227) -> (x*y=→"Trap 1 Position RMS (A)":dbl)
    n1752 = Divide(x=w2327, y=w2323) -> (x/y=w2295:waveform(dbl)[])
    n1753 = Index Array(array=w2295, index=0) -> (element=w2305:waveform(dbl))
    n1754 = case "For computing FFTs for display" shown="True" "Compute FFT" {
      tunnel: w2322 -> [_ w3425]
      frame False {
      }
      frame True {
        n1755 = Build Array("FFT 1 Choice 1", "FFT 1 Choice 2", "FFT 2 Choice 1", "FFT 2 Choice 2") -> (w3418:u16[])
        n1756 = Array Size(array=w3425) -> (size(s)=w3424:i32)
        n1757 = feedback-in #6(w3418) -> ()
        n1758 = feedback #6(u16[] [100, 100, 100, 100]) -> (w3419:u16[])
        n1759 = feedback-in #7("# Spectra to Ave.") -> ()
        n1760 = feedback #7("# Spectra to Ave.") -> (w3416:dbl)
        n1761 = Not Equal?(x="# Spectra to Ave.", y=w3416) -> (x != y?=w3415:bool)
        n1762 = Not Equal?(x=w3418, y=w3419) -> (x != y?=w3417:bool)
        n1763 = feedback #8(1.0) -> (w3402:dbl)
        n1764 = Compound Arithmetic op=OR("Reset FFT", w3417, w3415) -> (w3400:bool)
        n1765 = Select(t=1.0, s=w3400, f=w3402) -> (s? t:f=w3404:dbl)
        n1766 = Greater?(x=w3404, y="# Spectra to Ave.") -> (0:w3423:bool)
        n1767 = Increment(x=w3404) -> (x+1=w3403:dbl)
        n1768 = feedback-in #8(w3403) -> ()
        n1769 = local read "DMA Update Period (s)"() -> (w3398:dbl)
        n1770 = Multiply(x="# Spectra to Ave.", y=w3398) -> (x*y=→"Ave. Time (s)":dbl)
        n1771 = Build Array(cluster{"f0":dbl, "df":dbl, "magnitude":dbl[]} {"f0"=0.0, "df"=0.0, "magnitude"=[]} ("PSD")) -> (w3407:cluster{"f0":dbl, "df":dbl, "magnitude":dbl[]}[])
        n1772 = Build Array(w3407, w3407, w3407, w3407) -> (w3409:T47)
        n1773 = feedback #9(w3409) -> (w3414:T47)
        n1774 = for {
          N: 4 -> [_]
          tunnel: w3418 -> [w3447] mode=indexing
          tunnel: w3425 -> [w3448]
          tunnel: w3424 -> [w3450]
          tunnel: w3400 -> [w3443]
          tunnel: w3423 -> [w3442]
          tunnel: "# Spectra to Ave." -> [w3441]
          tunnel: [w3440] -> w3413 mode=indexing
          tunnel: w3414 -> [w3445] mode=indexing
          tunnel: [w3444] -> w3401 mode=indexing
          tunnel: w3404 -> [w3439]
          n1775 = Less?(x=w3447, y=w3450) -> (x < y?=w3449:bool)
          n1776 = Index Array(array=w3448, index=w3447) -> (element=w3446:waveform(dbl))
          n1777 = case shown="True" w3449 {
            tunnel: w3446 -> [_ w3467]
            tunnel: w3445 -> [w3452 w3465]
            tunnel: [w3452 w3453] -> w3444
            tunnel: w3443 -> [_ w3464]
            tunnel: w3442 -> [_ w3457]
            tunnel: w3441 -> [_ w3456]
            tunnel: [cluster{"f0":dbl, "df":dbl, "magnitude":dbl[]} {"f0"=0.0, "df"=0.0, "magnitude"=[]} ("PSD") w3458] -> w3440
            tunnel: w3439 -> [_ w3455]
            frame False {
            }
            frame True {
              n1778 = call <vilib>:"Std Deviation and Variance.vi"("X"=w3467) -> ("mean"=w3468:dbl)  [unwired: 1 in, 2 out]
              n1779 = Subtract(x=w3467, y=w3468) -> (x-y=w3466:waveform(dbl))
              n1780 = xnode "Spectral Measurements"("Signals"=w3466) -> ("PSD"=w3460:cluster{"f0":dbl, "df":dbl, "magnitude":dbl[]})  [unwired: 1 in, 1 out]
              n1781 = case shown="False" w3464 {
                tunnel: w3465 -> [w3477 _]
                tunnel: [w3473 w3482] -> w3453
                tunnel: w3460 -> [w3476 w3483]
                tunnel: w3457 -> [w3475 _]
                frame False {
                  n1782 = Build Array (concatenate)(w3477, w3476) -> (w3474:cluster{"f0":dbl, "df":dbl, "magnitude":dbl[]}[])
                  n1783 = case shown="True" w3475 {
                    tunnel: w3474 -> [w3478 w3481]
                    tunnel: [w3478 w3479] -> w3473
                    frame False {
                    }
                    frame True {
                      n1784 = Delete From Array(array=w3481, index=0) -> (array with subset deleted=w3479:cluster{"f0":dbl, "df":dbl, "magnitude":dbl[]}[])  [unwired: 1 in, 1 out]
                    }
                  }
                }
                frame True {
                  n1785 = Build Array(w3483) -> (w3482:cluster{"f0":dbl, "df":dbl, "magnitude":dbl[]}[])
                }
              }
              n1786 = for {
                tunnel: w3453 -> [w3472] mode=indexing
                tunnel: [w3471] -> w3463 mode=indexing
                workers-P: _ -> [_]
                n1787 = Unbundle By Name(w3472) -> ("magnitude"=w3471:dbl[])
              }
              n1788 = Transpose 2D Array(2D array=w3463) -> (transposed array=w3462:dbl[][])
              n1789 = for {
                tunnel: w3462 -> [w3470] mode=indexing
                tunnel: [w3469] -> w3461 mode=indexing
                workers-P: _ -> [_]
                n1790 = Add Array Elements(numeric array=w3470) -> (sum=w3469:dbl)
              }
              n1791 = Select(t=w3456, s=w3457, f=w3455) -> (s? t:f=w3454:dbl)
              n1792 = Divide(x=w3461, y=w3454) -> (x/y=w3459:dbl[])
              n1793 = Bundle By Name(cluster=w3460, "magnitude"=w3459) -> (w3458:cluster{"f0":dbl, "df":dbl, "magnitude":dbl[]})
            }
          }
        }
        n1794 = case shown="True" w3400 {
          tunnel: w3401 -> [w3432 w3438]
          tunnel: [w3432 w3433] -> w3399
          frame False {
          }
          frame True {
            n1795 = Array Subset(array=w3438, index (row)=0 ("index"), length (row)=4 ("length"), index (col)=0 ("index"), length (col)=1 ("length")) -> (w3433:T47)
          }
        }
        n1796 = feedback-in #9(w3399) -> ()
        n1797 = Split 1D Array(array=w3413, index=2) -> (first subarray=→"FFT 1":cluster{"f0":dbl, "df":dbl, "magnitude":dbl[]}[], second subarray=→"FFT 2":cluster{"f0":dbl, "df":dbl, "magnitude":dbl[]}[])
      }
    }
    n1798 = Index Array(array=w2295, index=1) -> (element=w2303:waveform(dbl))
    n1799 = case "For displaying the high resolution display (no downsampling)" shown="True" w2359 {
      tunnel: w2322 -> [_ w2641]
      frame False {
      }
      frame True {
        n1800 = Index Array(array=w2641, index="High Res. Display") -> (element=w2642:waveform(dbl))
        n1801 = call <vilib>:"Std Deviation and Variance.vi"("X"=w2642) -> ("mean"=w2649:dbl, "standard deviation"=w2654:dbl)  [unwired: 1 in, 1 out]
        "Mean Intensity" <- w2649
        "Sigma" <- w2654
        n1802 = Subtract(x=w2642, y=w2649) -> (x-y=w2648:waveform(dbl))
        n1803 = Select(t=w2648, s="Subtract mean", f=w2642) -> (s? t:f=→"1 Channel":waveform(dbl))
        n1804 = Divide(x=w2654, y=w2649) -> (x/y=→"Sigma/Mean":dbl)
        n1805 = feedback #10(1) -> (w2643:i32)
        n1806 = Greater Or Equal?(x=w2643, y="Slow mean N ave.") -> (x >= y?=w2656:bool)
        n1807 = Increment(x=w2643) -> (x+1=w2658:i32)
        n1808 = Select(t=1, s=w2656, f=w2658) -> (s? t:f=w2645:i32)
        n1809 = feedback-in #10(w2645) -> ()
        n1810 = feedback #11() -> (w2646:waveform(dbl))  [unwired: 1 out]
        n1811 = case shown="Default" w2643 {
          tunnel: [w2661 w2664] -> w2647
          tunnel: w2646 -> [w2663 _]
          tunnel: w2642 -> [w2662 w2664]
          frame Default {
            n1812 = call-poly <vilib>:"Append Waveforms.vi"("waveform B"=w2662, "waveform A"=w2663) -> ("waveform out"=w2661:waveform(dbl))  [unwired: 1 in, 8 out]
          }
          frame 1 {
          }
        }
        n1813 = feedback-in #11(w2647) -> ()
        n1814 = case shown="True" w2656 {
          tunnel: w2647 -> [_ w2660]
          frame False {
          }
          frame True {
            n1815 = call-poly <vilib>:"Mean.vi"("X"=w2660) -> ("mean"=→"Slow mean":dbl)  [unwired: 1 out]
          }
        }
      }
    }
    n1816 = case "For plotting results of scanning MCL" shown="True" w2429 {
      tunnel: w2428 -> [_ w2783]
      tunnel: w2352 -> [_ w2879]
      tunnel: w2437 -> [_ _]
      tunnel: w2322 -> [_ w2853]
      tunnel: w2297 -> [_ w2784]
      tunnel: w2296 -> [_ w2757]
      frame False {
      }
      frame True {
        w2764 = u32 0 items=["Horizontal", "Vertical", "Central", "1st Diagonal", "2nd Diagonal"] ("Type of Symmetry")
        w2792 = u32 0 items=["Horizontal", "Vertical", "Central", "1st Diagonal", "2nd Diagonal"] ("Type of Symmetry")
        w2795 = u32 0 items=["Horizontal", "Vertical", "Central", "1st Diagonal", "2nd Diagonal"] ("Type of Symmetry")
        w2824 = u32 0 items=["Horizontal", "Vertical", "Central", "1st Diagonal", "2nd Diagonal"] ("Type of Symmetry")
        n1817 = Index Array(array=w2853, index=10) -> (element=w2859:waveform(dbl))
        n1818 = Index Array(array=w2853, index=11) -> (element=w2856:waveform(dbl))
        n1819 = local read "Cycles/step (MCL)"() -> (w2809:u64)
        n1820 = Index Array(array=w2853, index="Channel") -> (element=w2855:waveform(dbl))
        n1821 = Unbundle(w2757) -> ("New Image"=w2756:T3, "New Image"=w2755:T3, "New Image"=w2754:T3, "New Image"=w2753:T3)
        n1822 = Unbundle By Name(w2859) -> ("Y"=w2811:dbl[])
        n1823 = Unbundle By Name(w2856) -> ("Y"=w2813:dbl[])
        n1824 = Unbundle By Name(w2855) -> ("Y"=w2818:dbl[])
        n1825 = call "downsample 1D array - double.vi"("Ave N"=w2809, "Array In"=w2811) -> ("Array Out"=w2810:dbl[])  [unwired: 1 out]
        n1826 = call "downsample 1D array - double.vi"("Ave N"=w2809, "Array In"=w2813) -> ("Array Out"=w2812:dbl[])  [unwired: 1 out]
        n1827 = call "downsample 1D array - double.vi"("Ave N"=w2809, "Array In"=w2818) -> ("Array Out"=w2817:dbl[])  [unwired: 1 out]
        n1828 = feedback #12(w2879) -> (w2880:dbl[])
        n1829 = Build Array (concatenate)(w2880, w2879) -> (w2861:dbl[])
        n1830 = feedback #13(w2784) -> (w2786:dbl[])
        n1831 = Build Array (concatenate)(w2786, w2784) -> (w2785:dbl[])
        n1832 = local read "Scan steps (MCL)"() -> (w2766:u64)
        n1833 = Select(t=w2879, s=w2783, f=w2861) -> (s? t:f=w2865:dbl[])
        n1834 = feedback-in #12(w2865) -> ()
        n1835 = Select(t=w2784, s=w2783, f=w2785) -> (s? t:f=w2767:dbl[])
        n1836 = feedback-in #13(w2767) -> ()
        n1837 = local read "Scan lines (y)"() -> (w2752:u64)
        n1838 = local read "N APD Samp/step"() -> (w2768:dbl)
        n1839 = feedback #14(w2810) -> (w2867:dbl[])
        n1840 = Build Array (concatenate)(w2867, w2810) -> (w2858:dbl[])
        n1841 = feedback #15(w2817) -> (w2877:dbl[])
        n1842 = Build Array (concatenate)(w2877, w2817) -> (w2876:dbl[])
        n1843 = feedback #16(w2812) -> (w2869:dbl[])
        n1844 = Build Array (concatenate)(w2869, w2812) -> (w2870:dbl[])
        n1845 = Select(t=w2810, s=w2783, f=w2858) -> (s? t:f=w2814:dbl[])
        n1846 = feedback-in #14(w2814) -> ()
        n1847 = Select(t=w2817, s=w2783, f=w2876) -> (s? t:f=w2816:dbl[])
        n1848 = feedback-in #15(w2816) -> ()
        n1849 = Select(t=w2812, s=w2783, f=w2870) -> (s? t:f=w2815:dbl[])
        n1850 = feedback-in #16(w2815) -> ()
        n1851 = Multiply(x=w2766, y=u64 2) -> (x*y=w2751:u64)
        n1852 = call "integrate 1D array interval - double.vi"("Ave N"=w2768, "Array In"=w2767) -> ("Array Out"=w2779:dbl[])  [unwired: 1 out]
        n1853 = call "integrate 1D array interval - double.vi"("Ave N"=w2768, "Array In"=w2865) -> ("Array Out"=w2864:dbl[])  [unwired: 1 out]
        n1854 = Array Size(array=w2779) -> (size(s)=w2780:i32)
        n1855 = Array Size(array=w2864) -> (size(s)=w2866:i32)
        n1856 = Multiply(x=w2752, y=w2751) -> (x*y=w2782:u64)
        n1857 = Multiply(x=w2752, y=w2751) -> (x*y=w2874:u64)
        n1858 = call-poly <vilib>:"Mean.vi"("X"=w2814) -> ("mean"=w2798:dbl)  [unwired: 1 out]
        n1859 = Subtract(x=w2782, y=w2780) -> (x-y=w2773:u64)
